vi "Update Status List.vi"(8 "error in (no error)":errorcluster, 10 "Status List":string[](array[string]), 11 "Chat Window UI Controller in":refnum<class "Chat Window UI Controller.lvclass">) -> (0 "error out":errorcluster, 3 "Chat Window UI Controller out":refnum<class "Chat Window UI Controller.lvclass">)   [LabVIEW 2018, in "Chat Window UI Controller.lvlib" / "Chat Window UI Controller.lvclass"]
uses:
  Chat Window UI Controller.lvclass
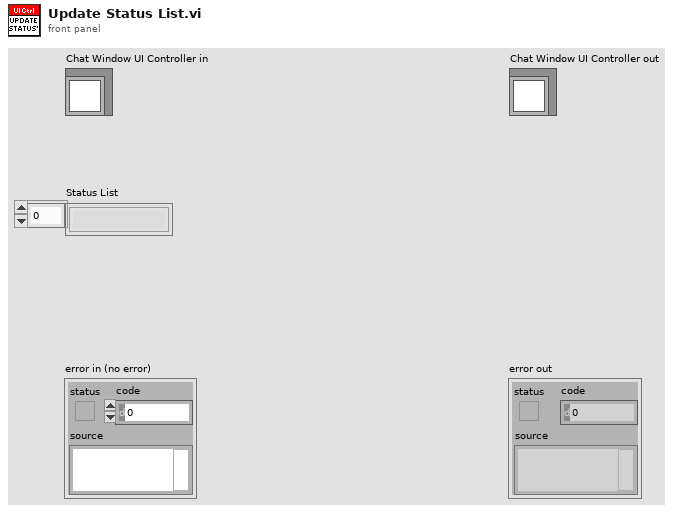
[diagram p1: front panel]
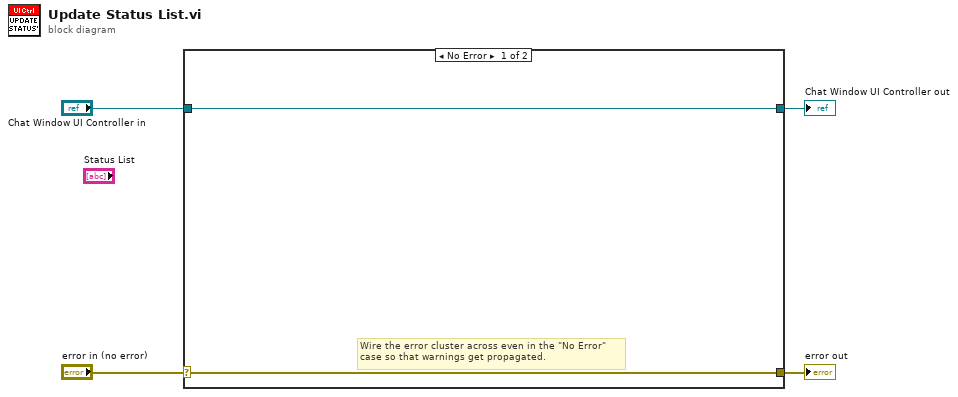
[diagram p0: block diagram]
diagram:
  n1 = case shown="No Error" "error in (no error)" {
    selector: "error in (no error)" -> [w5 w8]
    tunnel: [w5 w8] -> w3
    tunnel: [w6 w7] -> w1
    tunnel: "Chat Window UI Controller in" -> [w6 w7]
    frame No Error {
      # "Wire the error cluster across even in the \"No Error\"\ncase so that warnings get propagated."
    }
    frame Error {
    }
  }
  "error out" <- w3
  "Chat Window UI Controller out" <- w1
